vi "Autonomous Independent.vi"() -> ()   [LabVIEW 2013]
doc: "This VI is called when autonomous begins, and will automatically be terminated when autonomous ends. You can carry out timed or sensor driven robot movement independently without needing to return to the caller."
uses:
  <vilib>/Rock Robotics/WPI/RobotDrive/WPI_RobotDriveArcadeDrive_Standard(NoSaturation).vi
  Robot Global Data.vi
panel:
  out "Driving Dist":T1={"PID gains"={"proportional gain (Kc)"=1.0, "integral time (Ti, min)"=0.01, "derivative time (Td, min)"=0.0}, "output range"={"output high"=100.0, "output low"=-100.0}} {"output range"."output low" format="%.2f"; "output range"."output high" format="%.2f"; "PID gains"."derivative time (Td, min)" format="%.3f"; "PID gains"."integral time (Ti, min)" format="%.3f"; "PID gains"."proportional gain (Kc)" format="%.3f"}
  out "Current Movement, for debugging":T2 {"Y Joystick Value" scale=1.0..-1.0; "X Joystick Value" scale=-1.0..1.0}
  in  "Array of robot movements":T3(array[cluster]) {"Y Joystick Value" scale=1.0..-1.0; "X Joystick Value" scale=-1.0..1.0}
  # "Be sure to right-click and choose Data Operations>>Make Current Value default if you want to save the array values with the VI"
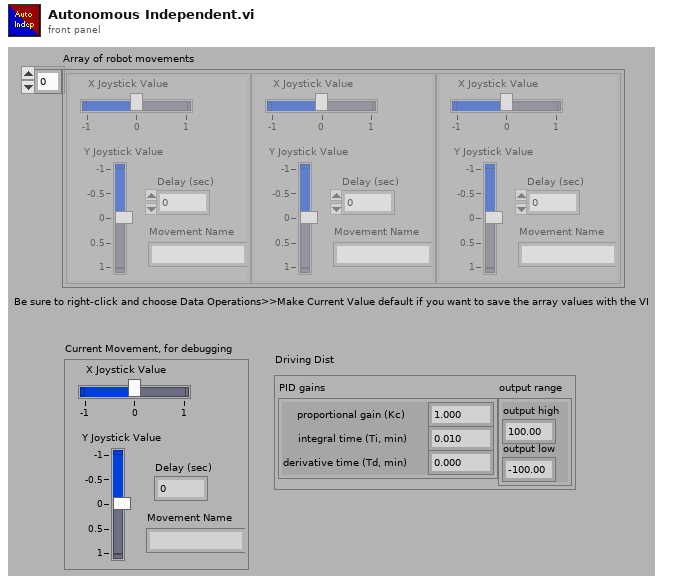
[diagram p1: front panel]
types:
  T1 = cluster{"PID gains":cluster{"proportional gain (Kc)":dbl, "integral time (Ti, min)":dbl, "derivative time (Td, min)":dbl}, "output range":cluster{"output high":dbl, "output low":dbl}}
  T2 = cluster{"X Joystick Value":dbl, "Y Joystick Value":dbl, "Delay (sec)":dbl, "Movement Name":string}
  T3 = cluster{"X Joystick Value":dbl, "Y Joystick Value":dbl, "Delay (sec)":dbl, "Movement Name":string}[]
  T4 = typedef "WPI_JoystickDevRef.ctl" = cluster{"Device":T5}
  T5 = typedef "WPI_JoystickDeviceEnum.ctl" = enum16{"USB 1", "USB 2", "USB 3", "USB 4", "Kinect 1", "Kinect 2"}
  T6 = cluster{"axis 1 (x)":dbl, "axis 2 (y)":dbl, "axis 3 (throttle)":dbl, "axis 4":dbl, "axis 5":dbl, "axis 6":dbl}
  T7 = typedef "WPI_RobotDriveDevRef.ctl" = cluster{"DevStatus":errorcluster, "Motors[]":T8[], "Square Inputs":bool, "Max Output":dbl, "Isochronous":bool}
  T8 = typedef "WPI_MotorControlDeviceRef.ctl" = cluster{"DeviceStatus":errorcluster, "Type":enum16{"PWM", "CAN"}, "PWM":cluster{"Digital Module":T9, "PWM Channel":T10, "DeadBand":T11}, "CAN":cluster{"Device Number":u8, "Control Mode":T12, "Semaphore":T13, "Max Vout":dbl}, "Invert":bool, "TransformRef":T14, "InvTransformRef":T14}
  T9 = typedef "FPGA_TypedefDigitalModule.ctl" = enum16{"Digital Module 1", "Digital Module 2"}
  T10 = typedef "FPGA_DIOPWMChannel.ctl" = enum8{"PWM 1", "PWM 2", "PWM 3", "PWM 4", "PWM 5", "PWM 6", "PWM 7", "PWM 8", "PWM 9", "PWM 10", "Invalid"}
  T11 = typedef "WPI_PWMDeadband.ctl" = cluster{"Name":string, "maxPositivePwm":i32, "minPositivePwm":i32, "centerPwm":i32, "maxNegativePwm":i32, "minNegativePwm":i32, "angularRange":u16}
  T12 = typedef "WPI_CANJaguar_ControlMode.ctl" = enum8{"Percent VBus", "Current", "Speed", "Position", "Voltage"}
  T13 = typedef "Semaphore RefNum" = refnum<k1>
  T14 = typedef "WPI_PWMTransform_ConPane.ctl" = refnum<vi>
  T15 = cluster{"proportional gain (Kc)":dbl, "integral time (Ti, min)":dbl, "derivative time (Td, min)":dbl}
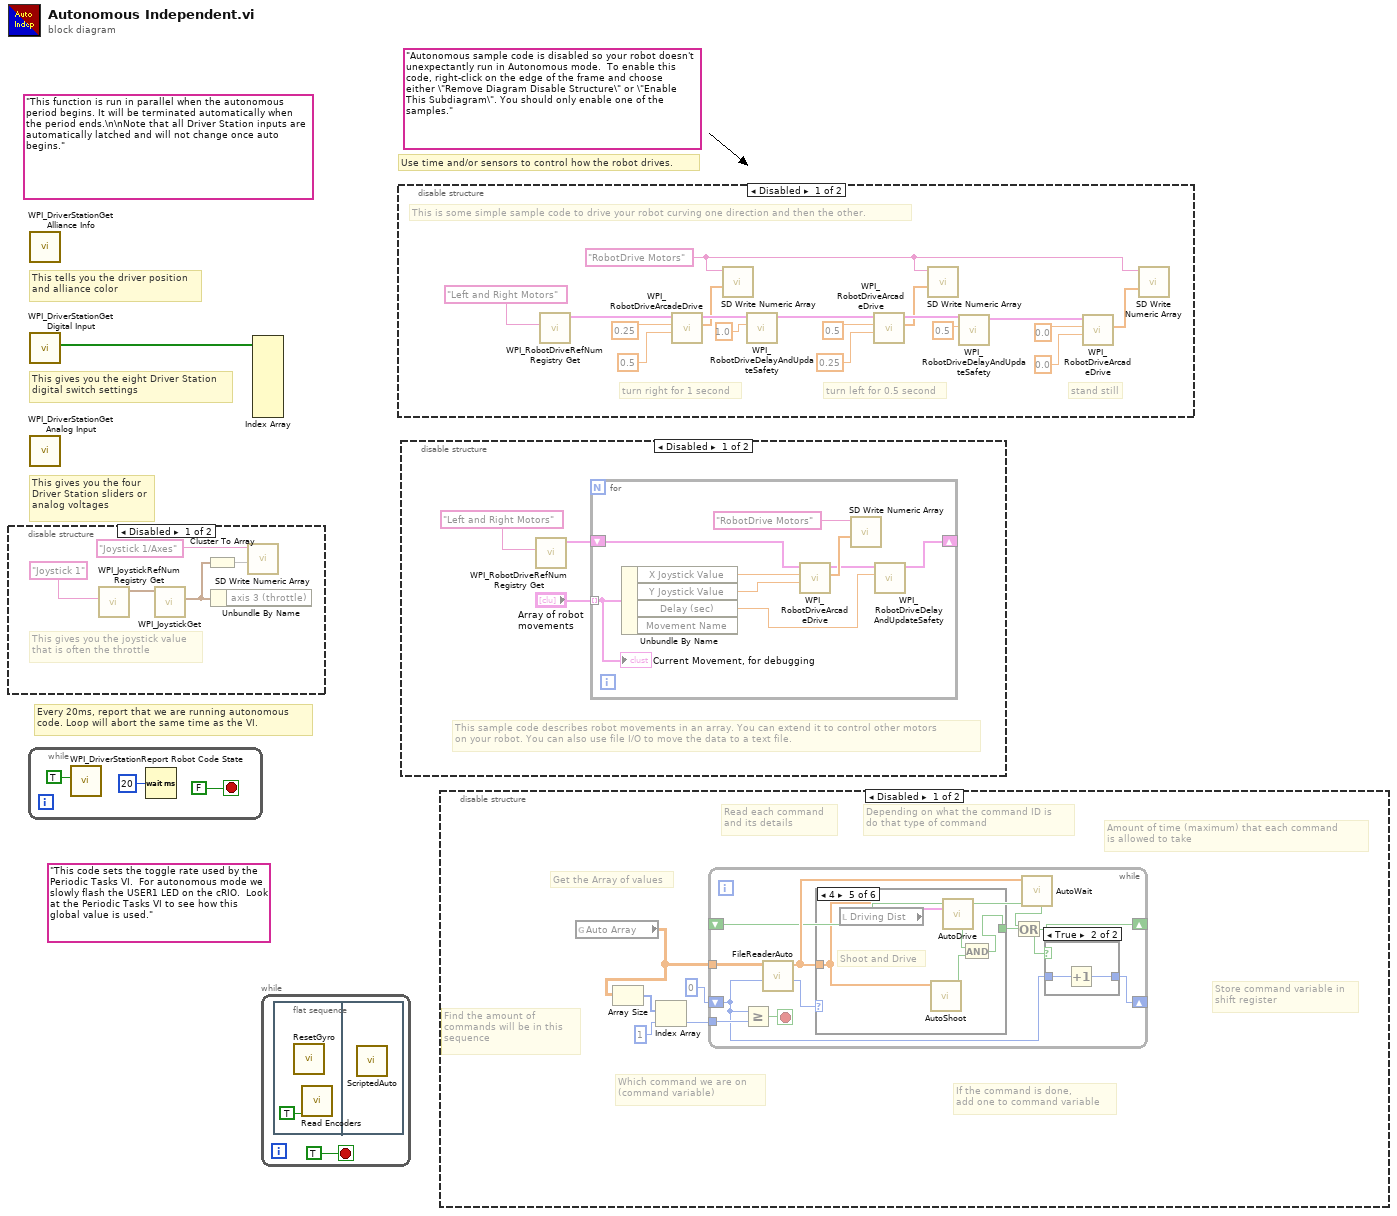
[diagram p0: block diagram]
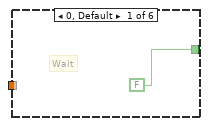
[diagram p3: hidden frame]
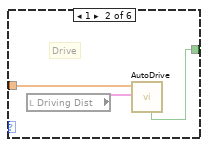
[diagram p4: hidden frame]
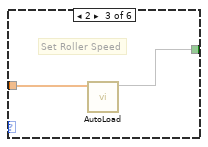
[diagram p5: hidden frame]
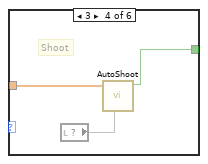
[diagram p6: hidden frame]
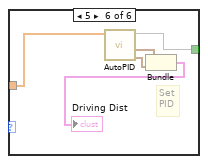
[diagram p7: hidden frame]
diagram:
  (unwired) "This code sets the toggle rate used by the Periodic Tasks VI.  For autonomous mode we slowly flash the USER1 LED on the cRIO.  Look at the Periodic Tasks VI to see how this global value is used."
  (unwired) "Autonomous sample code is disabled so your robot doesn't unexpectantly run in Autonomous mode.  To enable this code, right-click on the edge of the frame and choose either \"Remove Diagram Disable Structure\" or \"Enable This Subdiagram\". You should only enable one of the samples."
  (unwired) "This function is run in parallel when the autonomous period begins. It will be terminated automatically when the period ends.\n\nNote that all Driver Station inputs are automatically latched and will not change once auto begins."
  # "Every 20ms, report that we are running autonomous\ncode. Loop will abort the same time as the VI."
  # "Use time and/or sensors to control how the robot drives."
  # "This tells you the driver position\nand alliance color"
  # "This gives you the eight Driver Station\ndigital switch settings"
  # "This gives you the four\nDriver Station sliders or\nanalog voltages"
  n1 = disable-structure shown="Disabled" {
    frame Disabled {
      # "This gives you the joystick value\nthat is often the throttle"
      n2 = call <vilib>:"WPI_JoystickRefNum Registry Get.vi"("refnum name"="Joystick 1") -> ("JoystickDevRef"=w5:T4)  [unwired: 1 in, 9 out]
      n3 = call <vilib>:"WPI_JoystickGet.vi"("JoystickDevRef"=w5) -> ("Axes"=w3:T6)  [unwired: 1 in, 5 out]
      n4 = Cluster To Array(cluster=w3) -> (array=w4:dbl[])
      n5 = Unbundle By Name(w3) -> ()  [unwired: 1 out]
      n6 = call <vilib>:"SD Write Numeric Array.vi"("Numeric Array"=w4, "Name"="Joystick 1/Axes") -> ()  [unwired: 8 in, 2 out]
    }
    frame Enabled {
    }
  }
  n7 = while {
    stop <- FALSE stop-if-true
    n8 = call <vilib>:"WPI_DriverStationReport Robot Code State.vi"("Autonomous"=TRUE) -> ()  [unwired: 10 in, 1 out]
    n9 = Wait (ms)(milliseconds to wait=u32 20) -> ()  [unwired: 1 out]
  }
  n10 = call <vilib>:"WPI_DriverStationGet Alliance Info.vi"() -> ()  [unwired: 12 out]
  n11 = call <vilib>:"WPI_DriverStationGet Digital Input.vi"() -> ("Driver Station Digital Input (1-8)"=w1:bool[])  [unwired: 11 out]
  n12 = call <vilib>:"WPI_DriverStationGet Analog Input.vi"() -> ()  [unwired: 12 out]
  n13 = Index Array(array=w1) -> ()  [unwired: 8 in, 8 out]
  n14 = while {
    stop <- TRUE stop-if-true
    n15 = flat-sequence {
      frame #0 {
        n16 = call "ResetGyro.vi"() -> ()  [unwired: 12 in]
        n17 = call "Read Encoders.vi"("Reset"=TRUE) -> ()  [unwired: 10 in, 1 out]
      }
      frame #1 {
        n18 = call "ScriptedAuto.vi"() -> ()  [unwired: 12 in]
      }
    }
  }
  n19 = disable-structure shown="Disabled" {
    frame Disabled {
      w12 = "RobotDrive Motors" ("Name")
      # "This is some simple sample code to drive your robot curving one direction and then the other."
      # "stand still"
      # "turn left for 0.5 second"
      # "turn right for 1 second"
      n20 = call <vilib>:"WPI_RobotDriveRefNum Registry Get.vi"("refnum name"="Left and Right Motors") -> ("RobotDriveDevRef"=w16:T7)  [unwired: 1 in, 9 out]
      n21 = call-poly <vilib>:"WPI_RobotDriveArcadeDrive.vi"("Y axis value"=0.5 ("X axis value"), "X axis value"=0.25, "RobotDriveDevRef"=w16) -> ("Motor Values"=w15:dbl[], "RobotDriveDevRef"=w23:T7)  [unwired: 1 in, 6 out]
      n22 = call <vilib>:"SD Write Numeric Array.vi"("Numeric Array"=w15, "Name"=w12) -> ()  [unwired: 8 in, 2 out]
      n23 = call <vilib>:"WPI_RobotDriveDelayAndUpdateSafety.vi"("Delay (s)"=1.0, "RobotDriveDevRef"=w23) -> ("RobotDriveDevRef 2"=w22:T7)  [unwired: 8 in, 1 out]
      n24 = call-poly <vilib>:"WPI_RobotDriveArcadeDrive.vi"("Y axis value"=0.25 ("X axis value"), "X axis value"=0.5, "RobotDriveDevRef"=w22) -> ("Motor Values"=w14:dbl[], "RobotDriveDevRef"=w21:T7)  [unwired: 1 in, 6 out]
      n25 = call <vilib>:"SD Write Numeric Array.vi"("Numeric Array"=w14, "Name"=w12) -> ()  [unwired: 8 in, 2 out]
      n26 = call <vilib>:"WPI_RobotDriveDelayAndUpdateSafety.vi"("Delay (s)"=0.5, "RobotDriveDevRef"=w21) -> ("RobotDriveDevRef 2"=w20:T7)  [unwired: 8 in, 1 out]
      n27 = call-poly <vilib>:"WPI_RobotDriveArcadeDrive.vi"("Y axis value"=0.0 ("X axis value"), "X axis value"=0.0, "RobotDriveDevRef"=w20) -> ("Motor Values"=w13:dbl[])  [unwired: 1 in, 7 out]
      n28 = call <vilib>:"SD Write Numeric Array.vi"("Numeric Array"=w13, "Name"=w12) -> ()  [unwired: 8 in, 2 out]
    }
    frame Enabled {
    }
  }
  n29 = disable-structure shown="Disabled" {
    frame Disabled {
      # "This sample code describes robot movements in an array. You can extend it to control other motors\non your robot. You can also use file I/O to move the data to a text file."
      n30 = call <vilib>:"WPI_RobotDriveRefNum Registry Get.vi"("refnum name"="Left and Right Motors") -> ("RobotDriveDevRef"=w31:T7)  [unwired: 1 in, 9 out]
      n31 = for {
        shift-right: [w37] -> _
        shift-left: w31 -> [w38]
        tunnel: "Array of robot movements" -> [w33] mode=indexing
        n32 = Unbundle By Name(w33) -> ("X Joystick Value"=w36:dbl, "Y Joystick Value"=w35:dbl, "Delay (sec)"=w34:dbl)  [unwired: 1 out]
        n33 = call-poly <vilib>:"WPI_RobotDriveArcadeDrive.vi"("Y axis value"=w35, "X axis value"=w36, "RobotDriveDevRef"=w38) -> ("Motor Values"=w40:dbl[], "RobotDriveDevRef"=w39:T7)  [unwired: 1 in, 6 out]
        n34 = call <vilib>:"SD Write Numeric Array.vi"("Numeric Array"=w40, "Name"="RobotDrive Motors") -> ()  [unwired: 8 in, 2 out]
        n35 = call <vilib>:"WPI_RobotDriveDelayAndUpdateSafety.vi"("Delay (s)"=w34, "RobotDriveDevRef"=w39) -> ("RobotDriveDevRef 2"=w37:T7)  [unwired: 8 in, 1 out]
        "Current Movement, for debugging" <- w33
      }
    }
    frame Enabled {
    }
  }
  n36 = disable-structure shown="Disabled" {
    frame Disabled {
      # "Which command we are on\n(command variable)"
      # "Amount of time (maximum) that each command\nis allowed to take"
      # "If the command is done, \nadd one to command variable"
      # "Read each command\nand its details"
      # "Store command variable in\nshift register"
      # "Depending on what the command ID is\ndo that type of command"
      # "Get the Array of values"
      # "Find the amount of \ncommands will be in this \nsequence"
      n37 = global read "Robot Global Data.vi" "Auto Array"() -> (w42:dbl[][])
      n38 = Array Size(array=w42) -> (size(s)=w46:i32[])
      n39 = Index Array(array=w46, index=1) -> (element=w45:i32)
      n40 = while {
        tunnel: w42 -> [w49]
        tunnel: w45 -> [w57]
        shift-right: [w52] -> _
        shift-left: 0 -> [w55]
        shift-right: [w53] -> _
        shift-left: _ -> [w47]
        stop <- w56 stop-if-true
        n41 = Greater Or Equal?(x=w55, y=w57) -> (x >= y?=w56:bool)
        n42 = call "FileReaderAuto.vi"("index"=w55, "Auto Array"=w49) -> ("Command ID"=w51:i16, "Array"=w50:dbl[])  [unwired: 8 in]
        n43 = case shown="4" w51 {
          tunnel: w50 -> [_ w60 w62 w65 w70 w72]
          tunnel: [FALSE w61 w63 w66 w71 w73] -> w54
          frame 0, Default {
            # "Wait"
          }
          frame 1 {
            # "Drive"
            n44 = local read "Driving Dist"() -> (w59:T1)
            n45 = call "AutoDrive.vi"(9:w59, "Array"=w60) -> ("isFinished"=w61:bool)  [unwired: 9 in]
          }
          frame 2 {
            # "Set Roller Speed"
            n46 = call "AutoLoad.vi"("Array"=w62) -> (3:w63)  [unwired: 10 in]
          }
          frame 3 {
            # "Shoot"
            n47 = local read item#-1() -> (w64)
            n48 = call "AutoShoot.vi"(6:w64, "Array"=w65) -> ("isFinished"=w66:bool)  [unwired: 9 in]
          }
          frame 4 {
            # "Shoot and Drive"
            n49 = local read "Driving Dist"() -> (w68:T1)
            n50 = call "AutoShoot.vi"("Array"=w70) -> ("isFinished"=w67:bool)  [unwired: 10 in]
            n51 = call "AutoDrive.vi"(9:w68, "Array"=w70) -> ("isFinished"=w69:bool)  [unwired: 9 in]
            n52 = And(x=w69, y=w67) -> (x .and. y?=w71:bool)
          }
          frame 5 {
            # "Set \nPID"
            n53 = call "AutoPID.vi"("Array"=w72) -> ("output range"=w75:cluster{"output high":dbl, "output low":dbl}, "PID gains"=w74:T15, 3:w73)  [unwired: 8 in]
            n54 = Bundle("PID gains"=w74, "output range"=w75) -> (→"Driving Dist":T1)  [unwired: 1 in]
          }
        }
        n55 = call "AutoWait.vi"(8:w47, "Array"=w50) -> ("isFinished"=w48:bool)  [unwired: 9 in]
        n56 = Or(x=w48, y=w54) -> (x .or. y?=w53:bool)
        n57 = case shown="True" w53 {
          tunnel: w55 -> [w77 w79]
          tunnel: [w77 w78] -> w52
          frame False {
          }
          frame True {
            n58 = Increment(x=w79) -> (x+1=w78:i32)
          }
        }
      }
    }
    frame Enabled {
    }
  }
